vi "Prueba Trip Gap.vi"(11 "Class 2.lvclass":refnum<class "Class 2.lvclass">) -> (3 "Class 2.lvclass 2":refnum<class "Class 2.lvclass">)   [LabVIEW 2019, in "Class 2.lvclass"]
uses:
  Class 2.lvclass
  Class 2.lvclass/Class 2.ctl
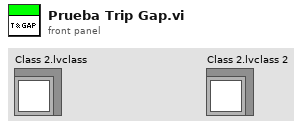
[diagram p1: front panel]
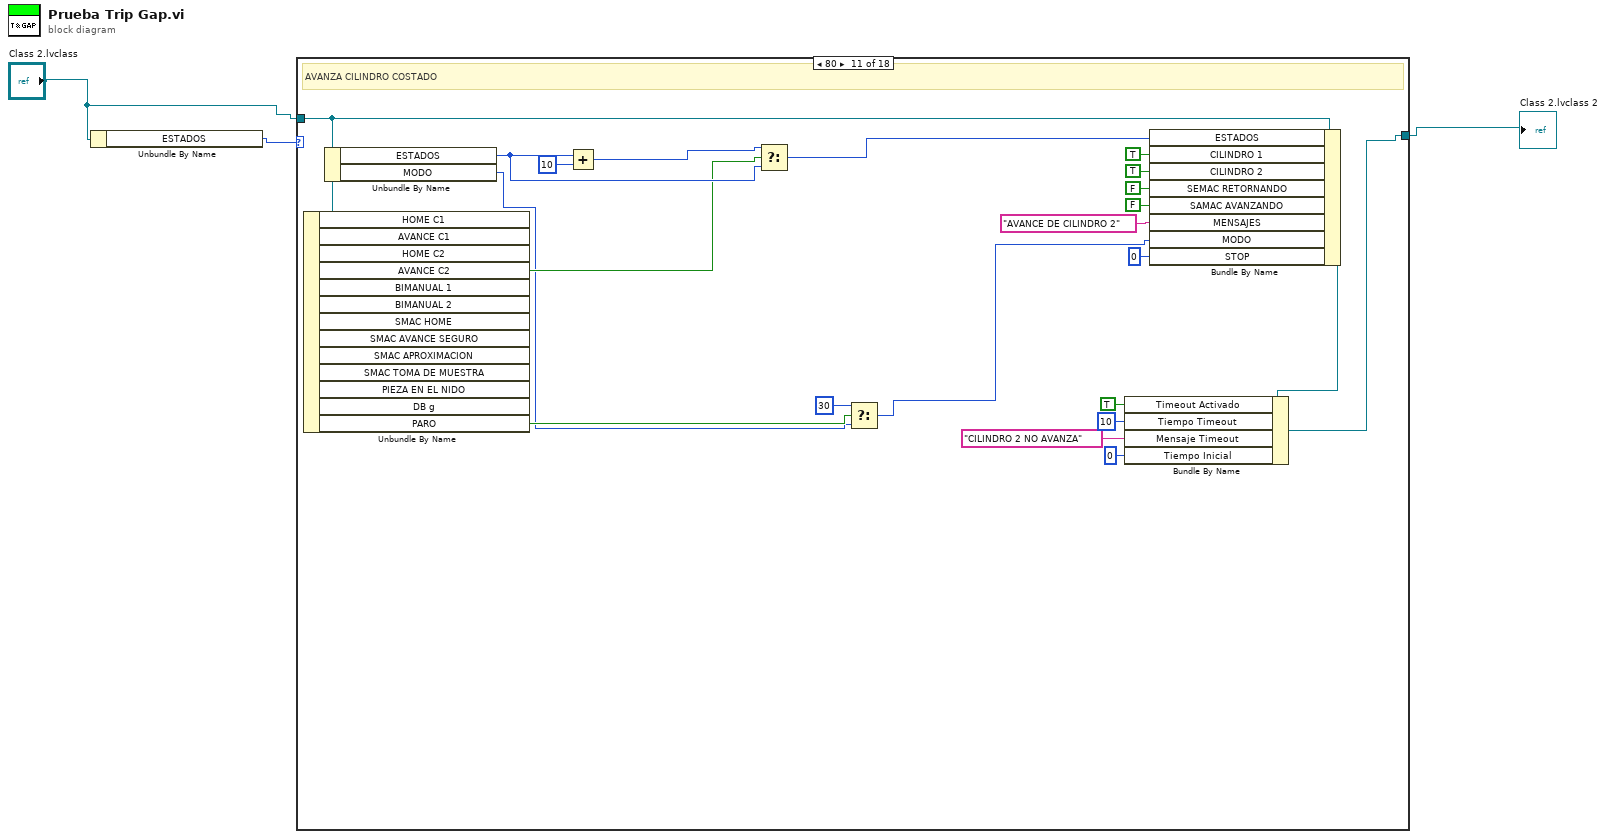
[diagram p0: block diagram]
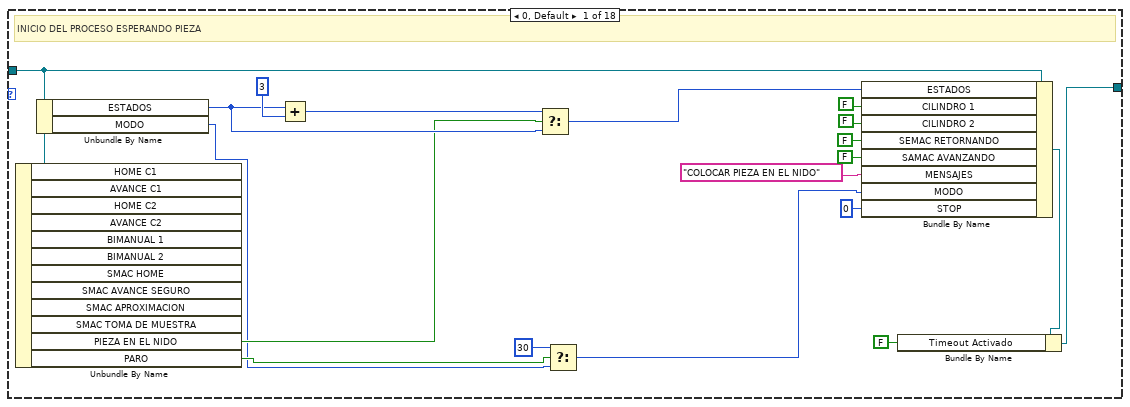
[diagram p2: hidden frame]
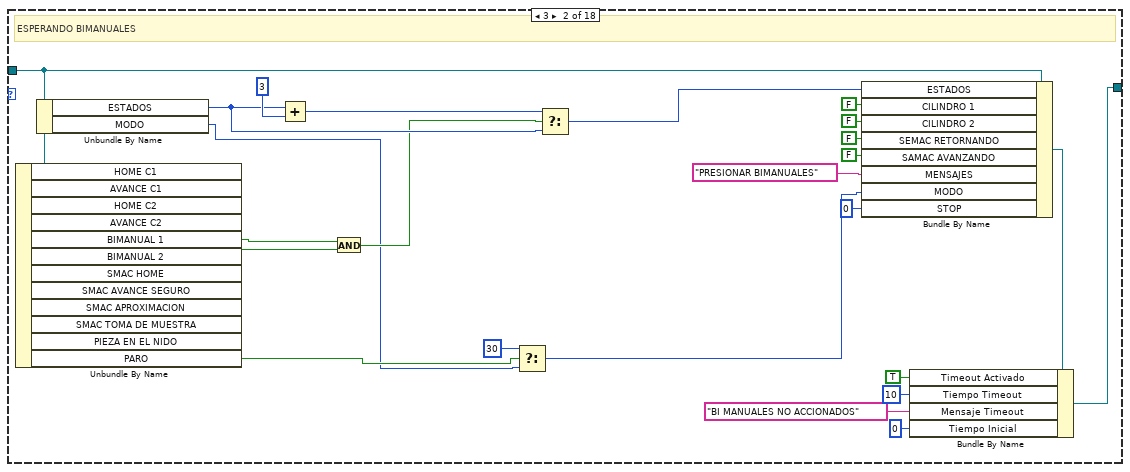
[diagram p3: hidden frame]
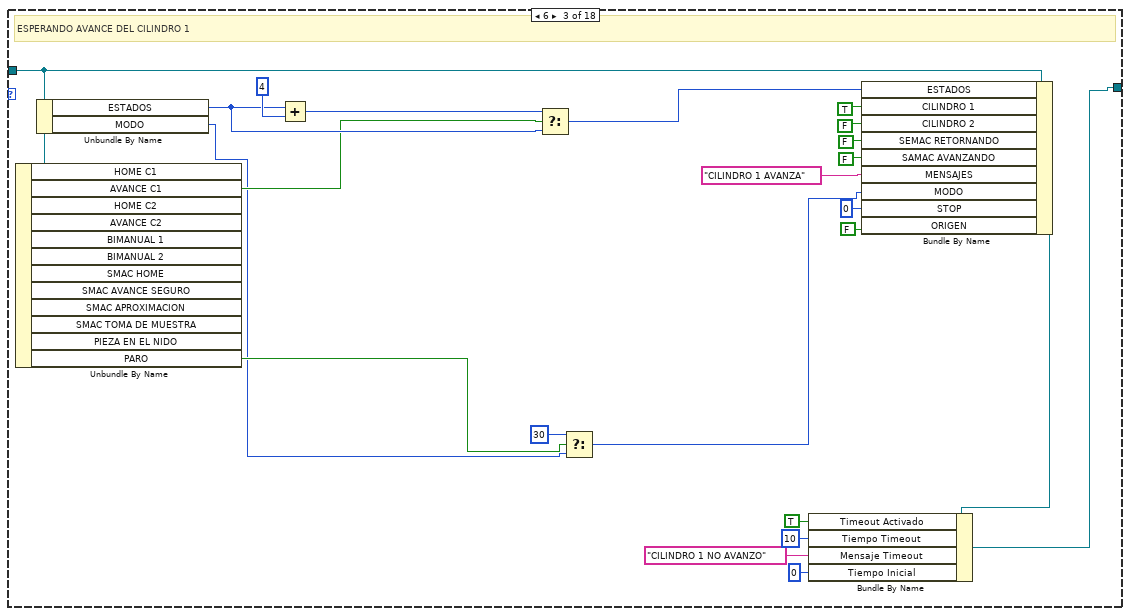
[diagram p4: hidden frame]
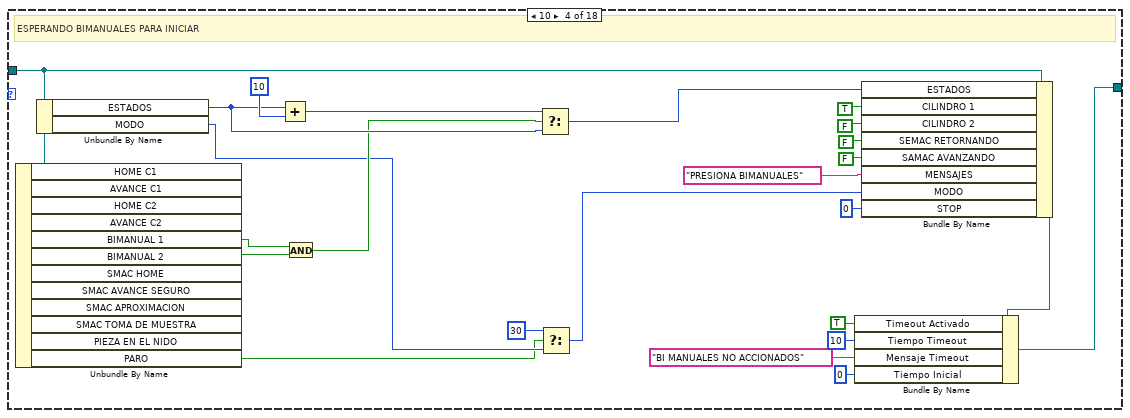
[diagram p5: hidden frame]
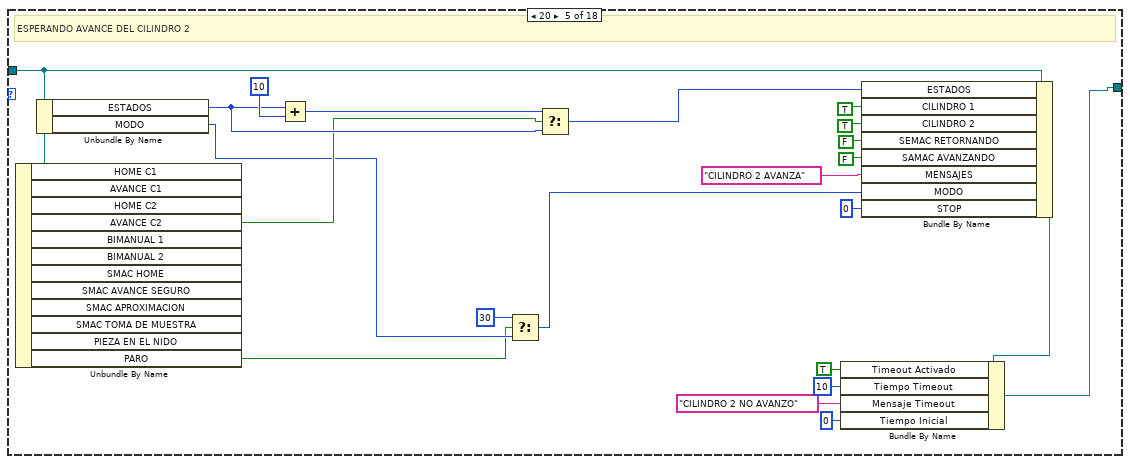
[diagram p6: hidden frame]
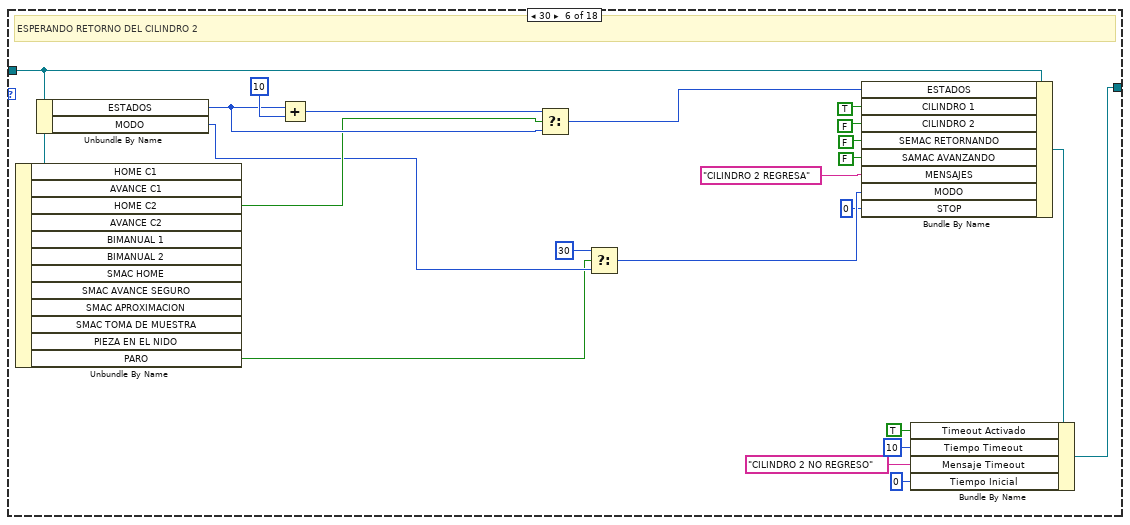
[diagram p7: hidden frame]
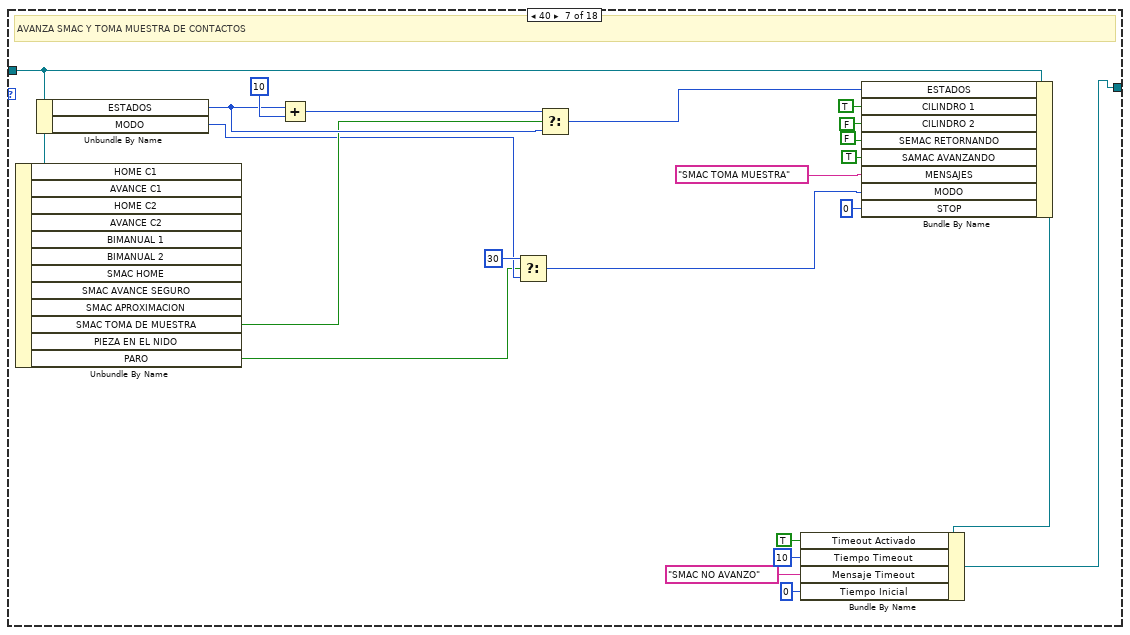
[diagram p8: hidden frame]
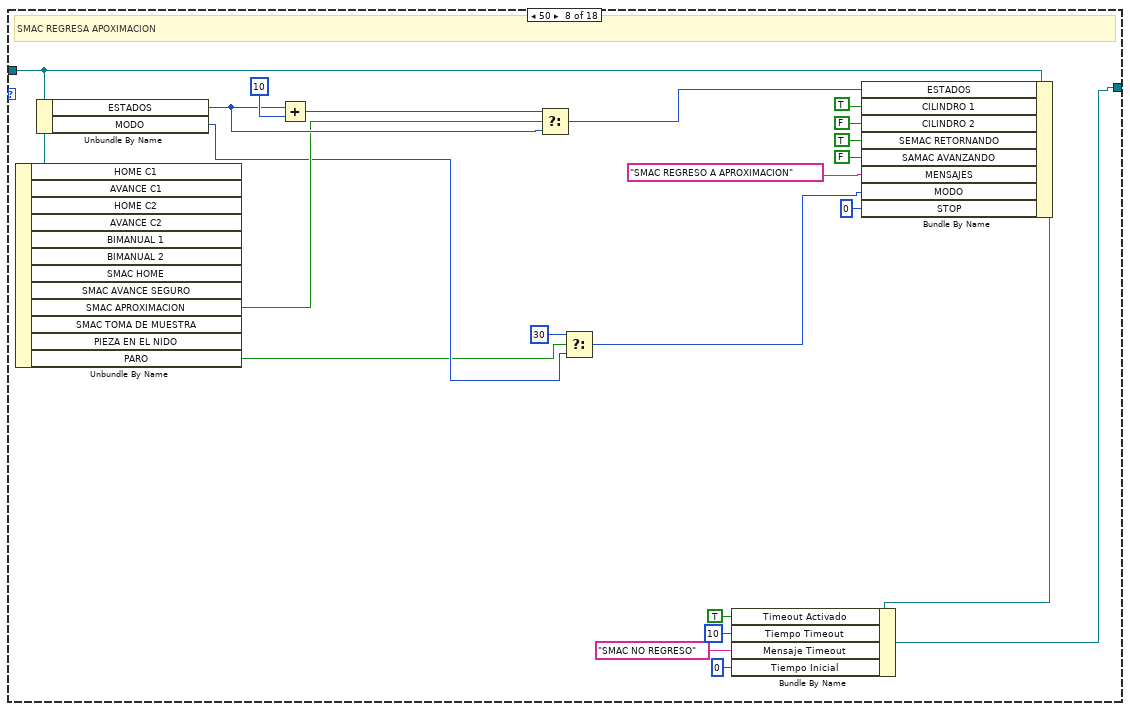
[diagram p9: hidden frame]
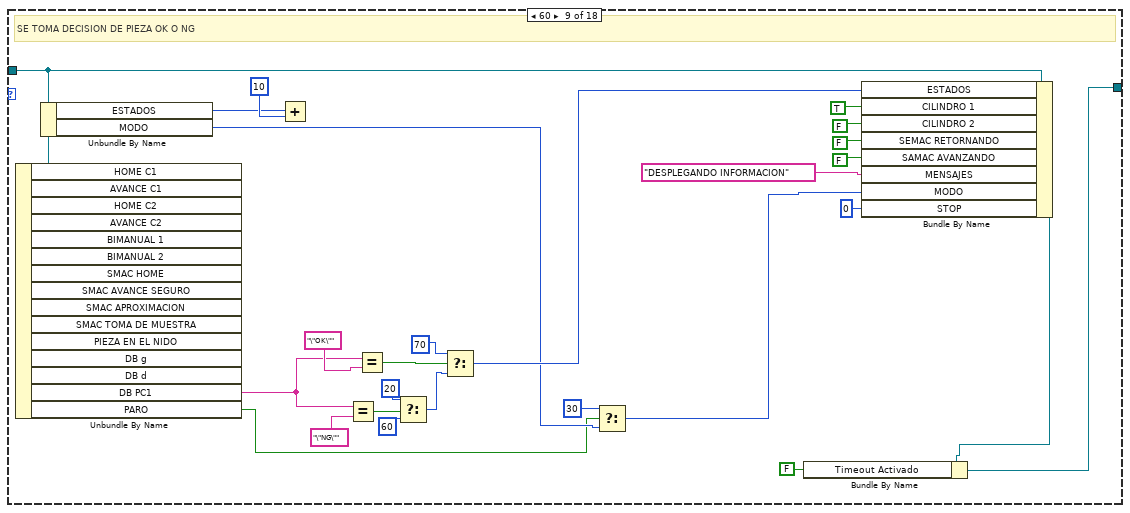
[diagram p10: hidden frame]
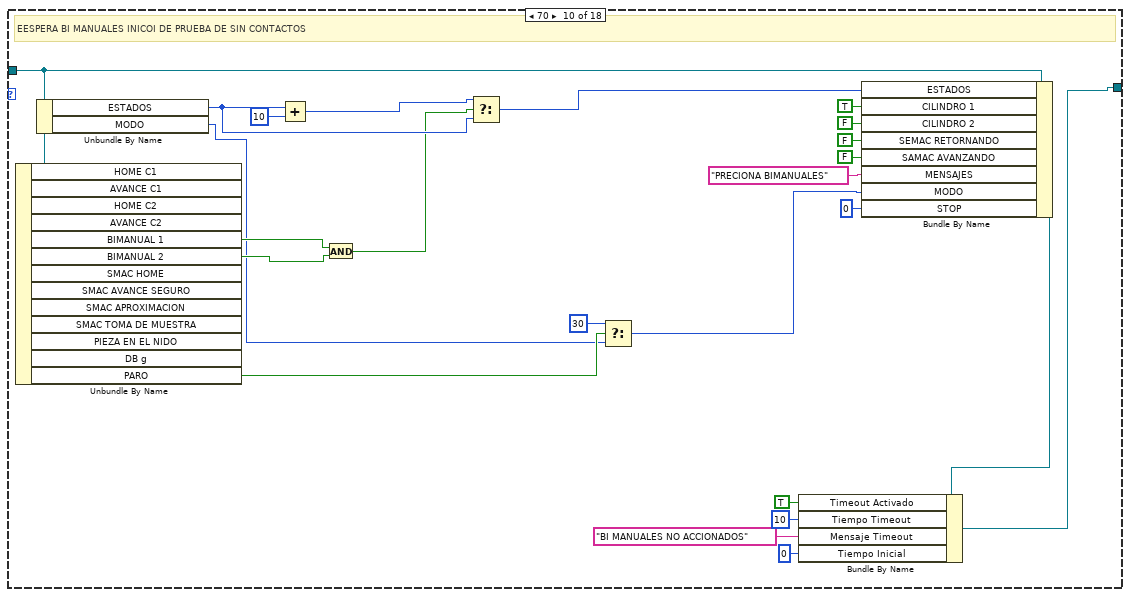
[diagram p11: hidden frame]
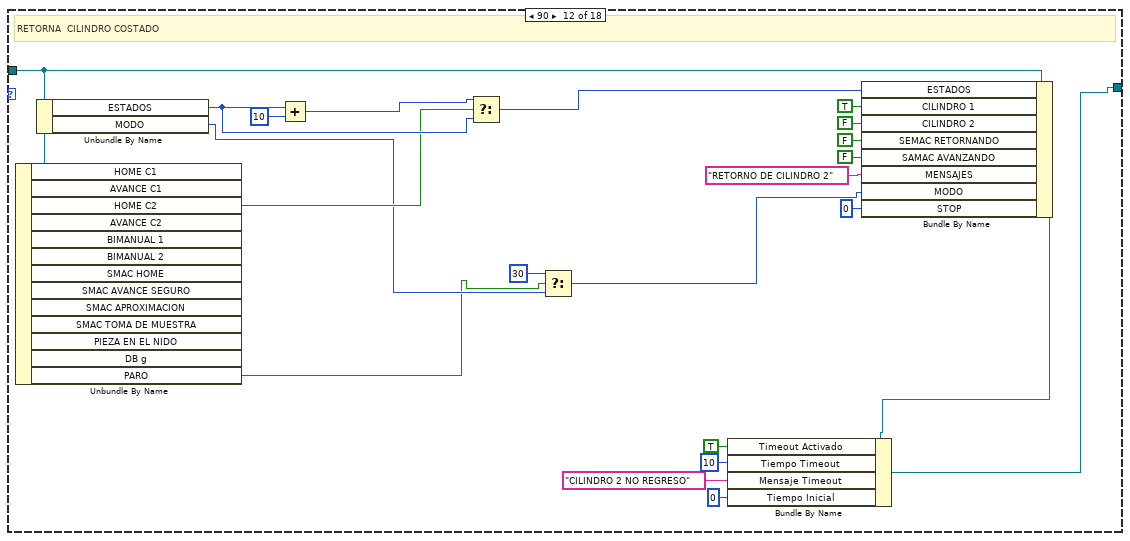
[diagram p12: hidden frame]
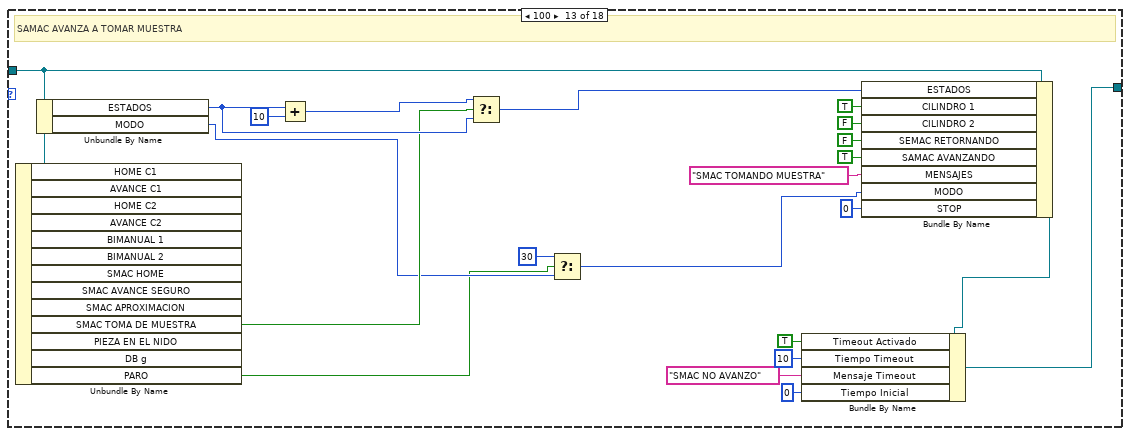
[diagram p13: hidden frame]
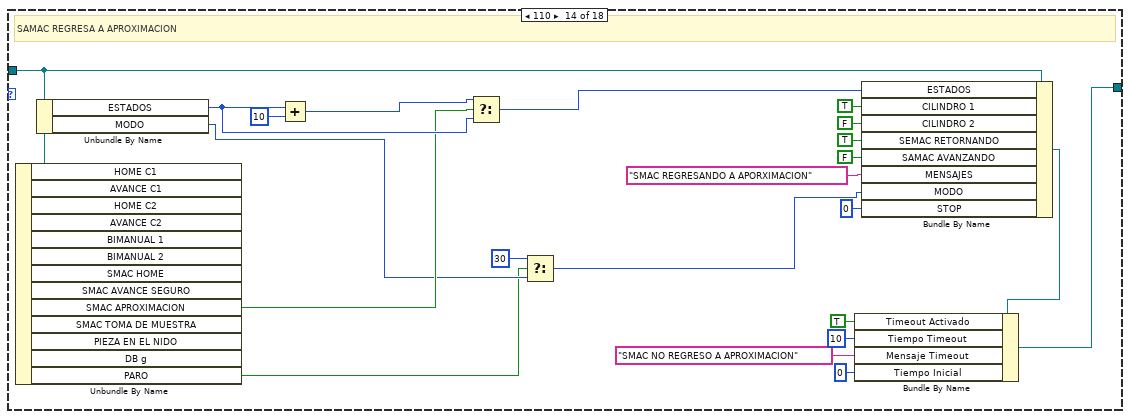
[diagram p14: hidden frame]
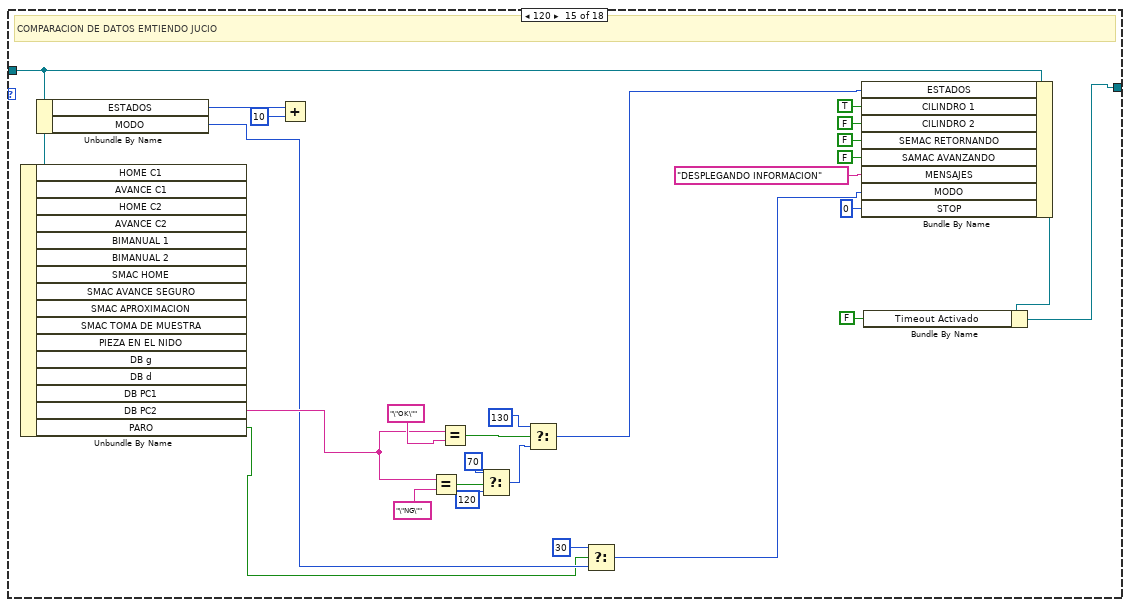
[diagram p15: hidden frame]
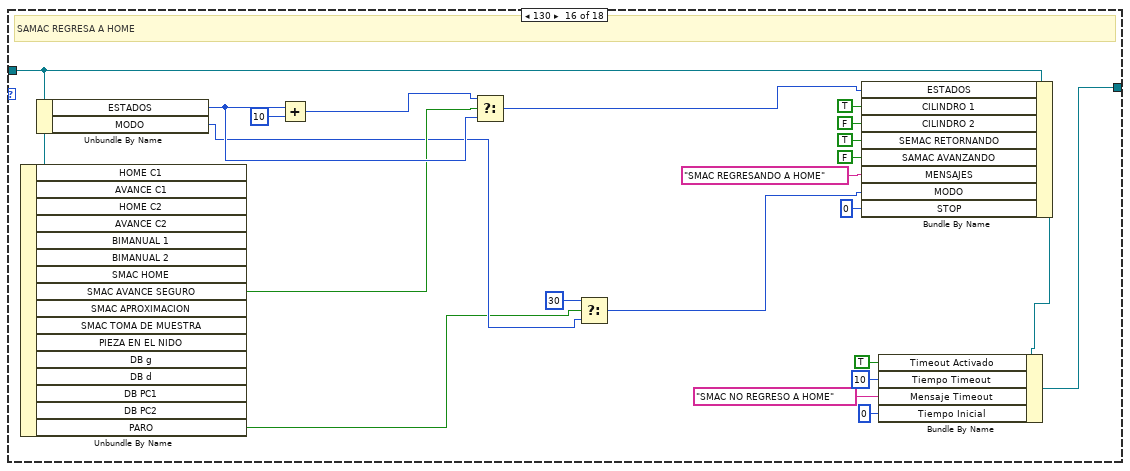
[diagram p16: hidden frame]
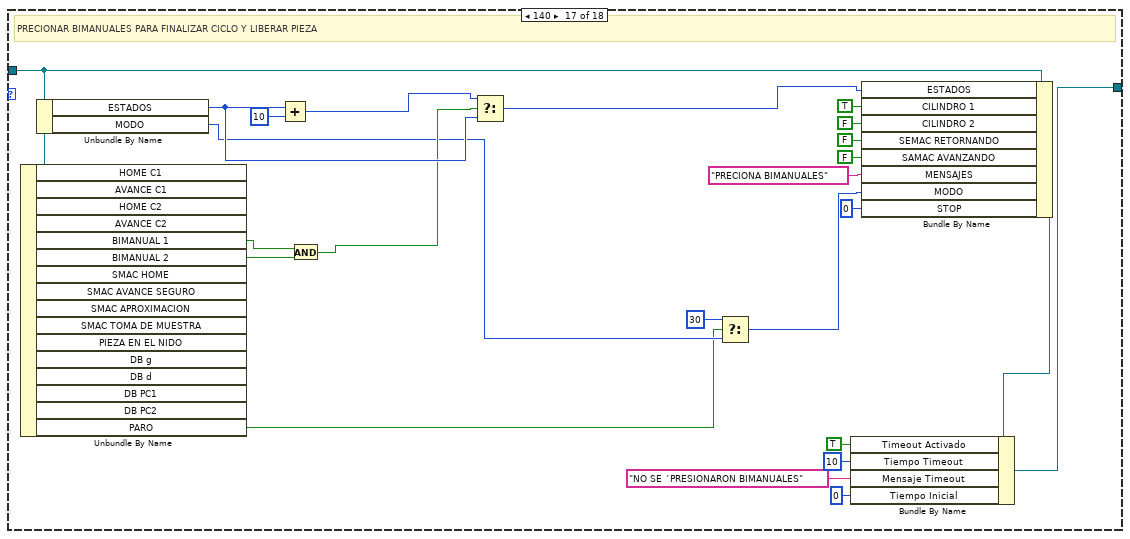
[diagram p17: hidden frame]
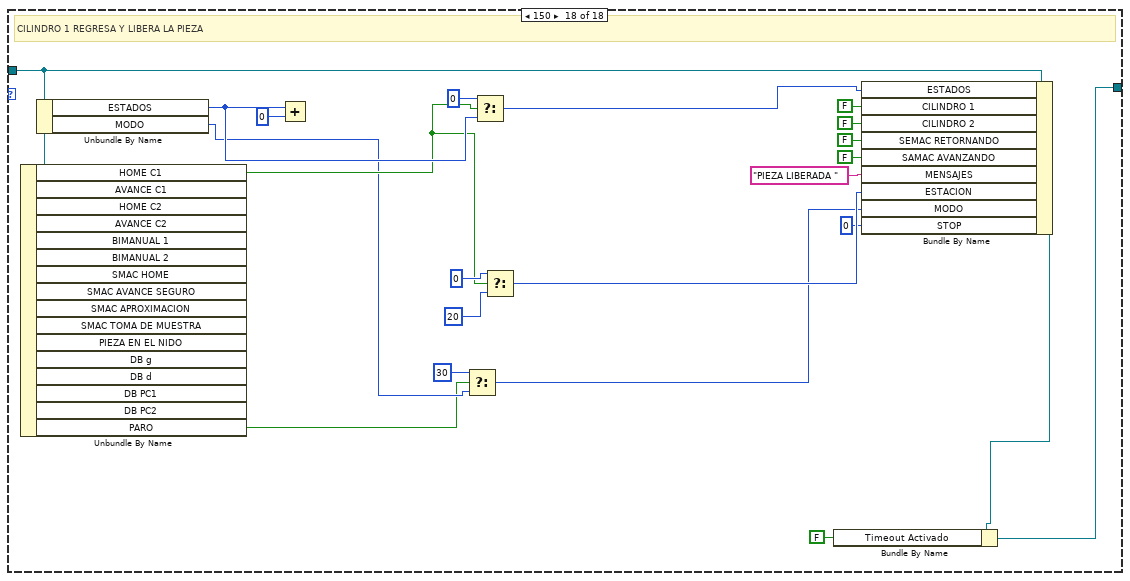
[diagram p18: hidden frame]
diagram:
  n1 = Unbundle By Name("Class 2.lvclass") -> ("ESTADOS"=w3:i16)
  n2 = case shown="80" w3 {
    tunnel: "Class 2.lvclass" -> [w18 w42 w65 w89 w111 w133 w155 w177 w206 w230 w252 w274 w296 w318 w344 w366 w390 w412]
    tunnel: [w4 w23 w47 w70 w94 w116 w138 w160 w182 w208 w232 w254 w276 w298 w320 w346 w368 w392] -> w1
    frame 0, Default {
      # "INICIO DEL PROCESO ESPERANDO PIEZA"
      n3 = Unbundle By Name(w18) -> ("PIEZA EN EL NIDO"=w16:bool, "PARO"=w8:bool)  [unwired: 10 out]
      n4 = Unbundle By Name(w18) -> ("ESTADOS"=w20:i16, "MODO"=w7:i16)
      n5 = Add(x=w20, y=i16 3) -> (x+y=w21:i16)
      n6 = Select(t=w21, s=w16, f=w20) -> (s? t:f=w19:i16)
      n7 = Select(t=i16 30, s=w8, f=w7) -> (s? t:f=w10:i16)
      n8 = Bundle By Name(cluster=w18, "ESTADOS"=w19, "CILINDRO 1"=FALSE ("SALIDAS.CILINDRO 1"), "CILINDRO 2"=FALSE ("SALIDAS.CILINDRO 2"), "SEMAC RETORNANDO"=FALSE ("SALIDAS.SEMAC RETORNANDO"), "SAMAC AVANZANDO"=FALSE ("SALIDAS.SAMAC AVANZANDO"), "MENSAJES"="COLOCAR PIEZA EN EL NIDO" ("SALIDAS.MENSAJES"), "MODO"=w10, "STOP"=i16 0 ("MAQ DE ESTADOS.STOP")) -> (w5:refnum<class "Class 2.lvclass">)
      n9 = Bundle By Name(cluster=w5, "Timeout Activado"=FALSE ("Timeout.Timeout Activado")) -> (w4:refnum<class "Class 2.lvclass">)
    }
    frame 3 {
      # "ESPERANDO BIMANUALES"
      n10 = Unbundle By Name(w42) -> ("BIMANUAL 1"=w36:bool, "BIMANUAL 2"=w35:bool, "PARO"=w30:bool)  [unwired: 9 out]
      n11 = Unbundle By Name(w42) -> ("ESTADOS"=w44:i16, "MODO"=w29:i16)
      n12 = Add(x=w44, y=i16 3) -> (x+y=w45:i16)
      n13 = And(x=w36, y=w35) -> (x .and. y?=w34:bool)
      n14 = Select(t=i16 30, s=w30, f=w29) -> (s? t:f=w32:i16)
      n15 = Select(t=w45, s=w34, f=w44) -> (s? t:f=w43:i16)
      n16 = Bundle By Name(cluster=w42, "ESTADOS"=w43, "CILINDRO 1"=FALSE ("SALIDAS.CILINDRO 1"), "CILINDRO 2"=FALSE ("SALIDAS.CILINDRO 2"), "SEMAC RETORNANDO"=FALSE ("SALIDAS.SEMAC RETORNANDO"), "SAMAC AVANZANDO"=FALSE ("SALIDAS.SAMAC AVANZANDO"), "MENSAJES"="PRESIONAR BIMANUALES" ("SALIDAS.MENSAJES"), "MODO"=w32, "STOP"=i16 0 ("MAQ DE ESTADOS.STOP")) -> (w24:refnum<class "Class 2.lvclass">)
      n17 = Bundle By Name(cluster=w24, "Timeout Activado"=TRUE ("Timeout.Timeout Activado"), "Tiempo Timeout"=u32 10 ("Timeout.Tiempo Timeout"), "Mensaje Timeout"="BI MANUALES NO ACCIONADOS" ("Timeout.Mensaje Timeout"), "Tiempo Inicial"=u32 0 ("Timeout.Tiempo Inicial")) -> (w23:refnum<class "Class 2.lvclass">)
    }
    frame 6 {
      # "ESPERANDO AVANCE DEL CILINDRO 1"
      n18 = Unbundle By Name(w65) -> ("AVANCE C1"=w59:bool, "PARO"=w55:bool)  [unwired: 10 out]
      n19 = Unbundle By Name(w65) -> ("ESTADOS"=w67:i16, "MODO"=w54:i16)
      n20 = Add(x=w67, y=i16 4) -> (x+y=w68:i16)
      n21 = Select(t=w68, s=w59, f=w67) -> (s? t:f=w66:i16)
      n22 = Select(t=i16 30, s=w55, f=w54) -> (s? t:f=w57:i16)
      n23 = Bundle By Name(cluster=w65, "ESTADOS"=w66, "CILINDRO 1"=TRUE ("SALIDAS.CILINDRO 1"), "CILINDRO 2"=FALSE ("SALIDAS.CILINDRO 2"), "SEMAC RETORNANDO"=FALSE ("SALIDAS.SEMAC RETORNANDO"), "SAMAC AVANZANDO"=FALSE ("SALIDAS.SAMAC AVANZANDO"), "MENSAJES"="CILINDRO 1 AVANZA" ("SALIDAS.MENSAJES"), "MODO"=w57, "STOP"=i16 0 ("MAQ DE ESTADOS.STOP"), "ORIGEN"=FALSE ("PROCESO.ORIGEN")) -> (w48:refnum<class "Class 2.lvclass">)
      n24 = Bundle By Name(cluster=w48, "Timeout Activado"=TRUE ("Timeout.Timeout Activado"), "Tiempo Timeout"=u32 10 ("Timeout.Tiempo Timeout"), "Mensaje Timeout"="CILINDRO 1 NO AVANZO" ("Timeout.Mensaje Timeout"), "Tiempo Inicial"=u32 0 ("Timeout.Tiempo Inicial")) -> (w47:refnum<class "Class 2.lvclass">)
    }
    frame 10 {
      # "ESPERANDO BIMANUALES PARA INICIAR"
      n25 = Unbundle By Name(w89) -> ("BIMANUAL 1"=w83:bool, "BIMANUAL 2"=w82:bool, "PARO"=w76:bool)  [unwired: 9 out]
      n26 = Unbundle By Name(w89) -> ("ESTADOS"=w91:i16, "MODO"=w77:i16)
      n27 = Add(x=w91, y=i16 10) -> (x+y=w92:i16)
      n28 = And(x=w83, y=w82) -> (x .and. y?=w81:bool)
      n29 = Select(t=w92, s=w81, f=w91) -> (s? t:f=w90:i16)
      n30 = Select(t=i16 30, s=w76, f=w77) -> (s? t:f=w79:i16)
      n31 = Bundle By Name(cluster=w89, "ESTADOS"=w90, "CILINDRO 1"=TRUE ("SALIDAS.CILINDRO 1"), "CILINDRO 2"=FALSE ("SALIDAS.CILINDRO 2"), "SEMAC RETORNANDO"=FALSE ("SALIDAS.SEMAC RETORNANDO"), "SAMAC AVANZANDO"=FALSE ("SALIDAS.SAMAC AVANZANDO"), "MENSAJES"="PRESIONA BIMANUALES" ("SALIDAS.MENSAJES"), "MODO"=w79, "STOP"=i16 0 ("MAQ DE ESTADOS.STOP")) -> (w71:refnum<class "Class 2.lvclass">)
      n32 = Bundle By Name(cluster=w71, "Timeout Activado"=TRUE ("Timeout.Timeout Activado"), "Tiempo Timeout"=u32 10 ("Timeout.Tiempo Timeout"), "Mensaje Timeout"="BI MANUALES NO ACCIONADOS" ("Timeout.Mensaje Timeout"), "Tiempo Inicial"=u32 0 ("Timeout.Tiempo Inicial")) -> (w70:refnum<class "Class 2.lvclass">)
    }
    frame 20 {
      # "ESPERANDO AVANCE DEL CILINDRO 2"
      n33 = Unbundle By Name(w111) -> ("AVANCE C2"=w105:bool, "PARO"=w100:bool)  [unwired: 10 out]
      n34 = Unbundle By Name(w111) -> ("ESTADOS"=w113:i16, "MODO"=w101:i16)
      n35 = Add(x=w113, y=i16 10) -> (x+y=w114:i16)
      n36 = Select(t=i16 30, s=w100, f=w101) -> (s? t:f=w103:i16)
      n37 = Select(t=w114, s=w105, f=w113) -> (s? t:f=w112:i16)
      n38 = Bundle By Name(cluster=w111, "ESTADOS"=w112, "CILINDRO 1"=TRUE ("SALIDAS.CILINDRO 1"), "CILINDRO 2"=TRUE ("SALIDAS.CILINDRO 2"), "SEMAC RETORNANDO"=FALSE ("SALIDAS.SEMAC RETORNANDO"), "SAMAC AVANZANDO"=FALSE ("SALIDAS.SAMAC AVANZANDO"), "MENSAJES"="CILINDRO 2 AVANZA" ("SALIDAS.MENSAJES"), "MODO"=w103, "STOP"=i16 0 ("MAQ DE ESTADOS.STOP")) -> (w95:refnum<class "Class 2.lvclass">)
      n39 = Bundle By Name(cluster=w95, "Timeout Activado"=TRUE ("Timeout.Timeout Activado"), "Tiempo Timeout"=u32 10 ("Timeout.Tiempo Timeout"), "Mensaje Timeout"="CILINDRO 2 NO AVANZO" ("Timeout.Mensaje Timeout"), "Tiempo Inicial"=u32 0 ("Timeout.Tiempo Inicial")) -> (w94:refnum<class "Class 2.lvclass">)
    }
    frame 30 {
      # "ESPERANDO RETORNO DEL CILINDRO 2"
      n40 = Unbundle By Name(w133) -> ("HOME C2"=w127:bool, "PARO"=w122:bool)  [unwired: 10 out]
      n41 = Unbundle By Name(w133) -> ("ESTADOS"=w135:i16, "MODO"=w123:i16)
      n42 = Add(x=w135, y=i16 10) -> (x+y=w136:i16)
      n43 = Select(t=w136, s=w127, f=w135) -> (s? t:f=w134:i16)
      n44 = Select(t=i16 30, s=w122, f=w123) -> (s? t:f=w125:i16)
      n45 = Bundle By Name(cluster=w133, "ESTADOS"=w134, "CILINDRO 1"=TRUE ("SALIDAS.CILINDRO 1"), "CILINDRO 2"=FALSE ("SALIDAS.CILINDRO 2"), "SEMAC RETORNANDO"=FALSE ("SALIDAS.SEMAC RETORNANDO"), "SAMAC AVANZANDO"=FALSE ("SALIDAS.SAMAC AVANZANDO"), "MENSAJES"="CILINDRO 2 REGRESA" ("SALIDAS.MENSAJES"), "MODO"=w125, "STOP"=i16 0 ("MAQ DE ESTADOS.STOP")) -> (w117:refnum<class "Class 2.lvclass">)
      n46 = Bundle By Name(cluster=w117, "Timeout Activado"=TRUE ("Timeout.Timeout Activado"), "Tiempo Timeout"=u32 10 ("Timeout.Tiempo Timeout"), "Mensaje Timeout"="CILINDRO 2 NO REGRESO" ("Timeout.Mensaje Timeout"), "Tiempo Inicial"=u32 0 ("Timeout.Tiempo Inicial")) -> (w116:refnum<class "Class 2.lvclass">)
    }
    frame 40 {
      # "AVANZA SMAC Y TOMA MUESTRA DE CONTACTOS"
      n47 = Unbundle By Name(w155) -> ("SMAC TOMA DE MUESTRA"=w149:bool, "PARO"=w144:bool)  [unwired: 10 out]
      n48 = Unbundle By Name(w155) -> ("ESTADOS"=w157:i16, "MODO"=w145:i16)
      n49 = Add(x=w157, y=i16 10) -> (x+y=w158:i16)
      n50 = Select(t=i16 30, s=w144, f=w145) -> (s? t:f=w147:i16)
      n51 = Select(t=w158, s=w149, f=w157) -> (s? t:f=w156:i16)
      n52 = Bundle By Name(cluster=w155, "ESTADOS"=w156, "CILINDRO 1"=TRUE ("SALIDAS.CILINDRO 1"), "CILINDRO 2"=FALSE ("SALIDAS.CILINDRO 2"), "SEMAC RETORNANDO"=FALSE ("SALIDAS.SEMAC RETORNANDO"), "SAMAC AVANZANDO"=TRUE ("SALIDAS.SAMAC AVANZANDO"), "MENSAJES"="SMAC TOMA MUESTRA" ("SALIDAS.MENSAJES"), "MODO"=w147, "STOP"=i16 0 ("MAQ DE ESTADOS.STOP")) -> (w139:refnum<class "Class 2.lvclass">)
      n53 = Bundle By Name(cluster=w139, "Timeout Activado"=TRUE ("Timeout.Timeout Activado"), "Tiempo Timeout"=u32 10 ("Timeout.Tiempo Timeout"), "Mensaje Timeout"="SMAC NO AVANZO" ("Timeout.Mensaje Timeout"), "Tiempo Inicial"=u32 0 ("Timeout.Tiempo Inicial")) -> (w138:refnum<class "Class 2.lvclass">)
    }
    frame 50 {
      # "SMAC REGRESA APOXIMACION"
      n54 = Unbundle By Name(w177) -> ("SMAC APROXIMACION"=w171:bool, "PARO"=w166:bool)  [unwired: 10 out]
      n55 = Unbundle By Name(w177) -> ("ESTADOS"=w179:i16, "MODO"=w167:i16)
      n56 = Add(x=w179, y=i16 10) -> (x+y=w180:i16)
      n57 = Select(t=w180, s=w171, f=w179) -> (s? t:f=w178:i16)
      n58 = Select(t=i16 30, s=w166, f=w167) -> (s? t:f=w169:i16)
      n59 = Bundle By Name(cluster=w177, "ESTADOS"=w178, "CILINDRO 1"=TRUE ("SALIDAS.CILINDRO 1"), "CILINDRO 2"=FALSE ("SALIDAS.CILINDRO 2"), "SEMAC RETORNANDO"=TRUE ("SALIDAS.SEMAC RETORNANDO"), "SAMAC AVANZANDO"=FALSE ("SALIDAS.SAMAC AVANZANDO"), "MENSAJES"="SMAC REGRESO A APROXIMACION" ("SALIDAS.MENSAJES"), "MODO"=w169, "STOP"=i16 0 ("MAQ DE ESTADOS.STOP")) -> (w161:refnum<class "Class 2.lvclass">)
      n60 = Bundle By Name(cluster=w161, "Timeout Activado"=TRUE ("Timeout.Timeout Activado"), "Tiempo Timeout"=u32 10 ("Timeout.Tiempo Timeout"), "Mensaje Timeout"="SMAC NO REGRESO" ("Timeout.Mensaje Timeout"), "Tiempo Inicial"=u32 0 ("Timeout.Tiempo Inicial")) -> (w160:refnum<class "Class 2.lvclass">)
    }
    frame 60 {
      # "SE TOMA DECISION DE PIEZA OK O NG"
      n61 = Unbundle By Name(w206) -> ("DB PC1"=w190:string, "PARO"=w185:bool)  [unwired: 13 out]
      n62 = Unbundle By Name(w206) -> ("ESTADOS"=w199:i16, "MODO"=w186:i16)
      n63 = Add(x=w199, y=i16 10) -> ()  [unwired: 1 out]
      n64 = Equal?(x=w190, y="\"NG\"") -> (x = y?=w197:bool)
      n65 = Equal?(x=w190, y="\"OK\"") -> (x = y?=w198:bool)
      n66 = Select(t=i16 20 ("y"), s=w197, f=i16 60) -> (s? t:f=w194:i16)
      n67 = Select(t=i16 70, s=w198, f=w194) -> (s? t:f=w192:i16)
      n68 = Select(t=i16 30, s=w185, f=w186) -> (s? t:f=w188:i16)
      n69 = Bundle By Name(cluster=w206, "ESTADOS"=w192, "CILINDRO 1"=TRUE ("SALIDAS.CILINDRO 1"), "CILINDRO 2"=FALSE ("SALIDAS.CILINDRO 2"), "SEMAC RETORNANDO"=FALSE ("SALIDAS.SEMAC RETORNANDO"), "SAMAC AVANZANDO"=FALSE ("SALIDAS.SAMAC AVANZANDO"), "MENSAJES"="DESPLEGANDO INFORMACION" ("SALIDAS.MENSAJES"), "MODO"=w188, "STOP"=i16 0 ("MAQ DE ESTADOS.MODO")) -> (w183:refnum<class "Class 2.lvclass">)
      n70 = Bundle By Name(cluster=w183, "Timeout Activado"=FALSE ("Timeout.Timeout Activado")) -> (w182:refnum<class "Class 2.lvclass">)
    }
    frame 70 {
      # "EESPERA BI MANUALES INICOI DE PRUEBA DE SIN CONTACTOS"
      n71 = Unbundle By Name(w230) -> ("BIMANUAL 1"=w221:bool, "BIMANUAL 2"=w220:bool, "PARO"=w217:bool)  [unwired: 10 out]
      n72 = Unbundle By Name(w230) -> ("ESTADOS"=w223:i16, "MODO"=w216:i16)
      n73 = Add(x=w223, y=i16 10) -> (x+y=w222:i16)
      n74 = And(x=w221, y=w220) -> (x .and. y?=w219:bool)
      n75 = Select(t=w222, s=w219, f=w223) -> (s? t:f=w224:i16)
      n76 = Select(t=i16 30, s=w217, f=w216) -> (s? t:f=w215:i16)
      n77 = Bundle By Name(cluster=w230, "ESTADOS"=w224, "CILINDRO 1"=TRUE ("SALIDAS.CILINDRO 1"), "CILINDRO 2"=FALSE ("SALIDAS.CILINDRO 2"), "SEMAC RETORNANDO"=FALSE ("SALIDAS.SEMAC RETORNANDO"), "SAMAC AVANZANDO"=FALSE ("SALIDAS.SAMAC AVANZANDO"), "MENSAJES"="PRECIONA BIMANUALES" ("SALIDAS.MENSAJES"), "MODO"=w215, "STOP"=i16 0 ("MAQ DE ESTADOS.STOP")) -> (w209:refnum<class "Class 2.lvclass">)
      n78 = Bundle By Name(cluster=w209, "Timeout Activado"=TRUE ("Timeout.Timeout Activado"), "Tiempo Timeout"=u32 10 ("Timeout.Tiempo Timeout"), "Mensaje Timeout"="BI MANUALES NO ACCIONADOS" ("Timeout.Mensaje Timeout"), "Tiempo Inicial"=u32 0 ("Timeout.Tiempo Inicial")) -> (w208:refnum<class "Class 2.lvclass">)
    }
    frame 80 {
      # "AVANZA CILINDRO COSTADO"
      n79 = Unbundle By Name(w252) -> ("AVANCE C2"=w243:bool, "PARO"=w241:bool)  [unwired: 11 out]
      n80 = Unbundle By Name(w252) -> ("ESTADOS"=w245:i16, "MODO"=w240:i16)
      n81 = Add(x=w245, y=i16 10) -> (x+y=w244:i16)
      n82 = Select(t=w244, s=w243, f=w245) -> (s? t:f=w246:i16)
      n83 = Select(t=i16 30, s=w241, f=w240) -> (s? t:f=w239:i16)
      n84 = Bundle By Name(cluster=w252, "ESTADOS"=w246, "CILINDRO 1"=TRUE ("SALIDAS.CILINDRO 1"), "CILINDRO 2"=TRUE ("SALIDAS.CILINDRO 2"), "SEMAC RETORNANDO"=FALSE ("SALIDAS.SEMAC RETORNANDO"), "SAMAC AVANZANDO"=FALSE ("SALIDAS.SAMAC AVANZANDO"), "MENSAJES"="AVANCE DE CILINDRO 2" ("SALIDAS.MENSAJES"), "MODO"=w239, "STOP"=i16 0 ("MAQ DE ESTADOS.STOP")) -> (w233:refnum<class "Class 2.lvclass">)
      n85 = Bundle By Name(cluster=w233, "Timeout Activado"=TRUE ("Timeout.Timeout Activado"), "Tiempo Timeout"=u32 10 ("Timeout.Tiempo Timeout"), "Mensaje Timeout"="CILINDRO 2 NO AVANZA" ("Timeout.Mensaje Timeout"), "Tiempo Inicial"=u32 0 ("Timeout.Tiempo Inicial")) -> (w232:refnum<class "Class 2.lvclass">)
    }
    frame 90 {
      # "RETORNA  CILINDRO COSTADO"
      n86 = Unbundle By Name(w274) -> ("HOME C2"=w265:bool, "PARO"=w261:bool)  [unwired: 11 out]
      n87 = Unbundle By Name(w274) -> ("ESTADOS"=w267:i16, "MODO"=w262:i16)
      n88 = Add(x=w267, y=i16 10) -> (x+y=w266:i16)
      n89 = Select(t=w266, s=w265, f=w267) -> (s? t:f=w268:i16)
      n90 = Select(t=i16 30, s=w261, f=w262) -> (s? t:f=w263:i16)
      n91 = Bundle By Name(cluster=w274, "ESTADOS"=w268, "CILINDRO 1"=TRUE ("SALIDAS.CILINDRO 1"), "CILINDRO 2"=FALSE ("SALIDAS.CILINDRO 2"), "SEMAC RETORNANDO"=FALSE ("SALIDAS.SEMAC RETORNANDO"), "SAMAC AVANZANDO"=FALSE ("SALIDAS.SAMAC AVANZANDO"), "MENSAJES"="RETORNO DE CILINDRO 2" ("SALIDAS.MENSAJES"), "MODO"=w263, "STOP"=i16 0 ("MAQ DE ESTADOS.STOP")) -> (w255:refnum<class "Class 2.lvclass">)
      n92 = Bundle By Name(cluster=w255, "Timeout Activado"=TRUE ("Timeout.Timeout Activado"), "Tiempo Timeout"=u32 10 ("Timeout.Tiempo Timeout"), "Mensaje Timeout"="CILINDRO 2 NO REGRESO" ("Timeout.Mensaje Timeout"), "Tiempo Inicial"=u32 0 ("Timeout.Tiempo Inicial")) -> (w254:refnum<class "Class 2.lvclass">)
    }
    frame 100 {
      # "SAMAC AVANZA A TOMAR MUESTRA"
      n93 = Unbundle By Name(w296) -> ("SMAC TOMA DE MUESTRA"=w287:bool, "PARO"=w282:bool)  [unwired: 11 out]
      n94 = Unbundle By Name(w296) -> ("ESTADOS"=w289:i16, "MODO"=w283:i16)
      n95 = Add(x=w289, y=i16 10) -> (x+y=w288:i16)
      n96 = Select(t=w288, s=w287, f=w289) -> (s? t:f=w290:i16)
      n97 = Select(t=i16 30, s=w282, f=w283) -> (s? t:f=w285:i16)
      n98 = Bundle By Name(cluster=w296, "ESTADOS"=w290, "CILINDRO 1"=TRUE ("SALIDAS.CILINDRO 1"), "CILINDRO 2"=FALSE ("SALIDAS.CILINDRO 2"), "SEMAC RETORNANDO"=FALSE ("SALIDAS.SEMAC RETORNANDO"), "SAMAC AVANZANDO"=TRUE ("SALIDAS.SAMAC AVANZANDO"), "MENSAJES"="SMAC TOMANDO MUESTRA" ("SALIDAS.MENSAJES"), "MODO"=w285, "STOP"=i16 0 ("MAQ DE ESTADOS.STOP")) -> (w277:refnum<class "Class 2.lvclass">)
      n99 = Bundle By Name(cluster=w277, "Timeout Activado"=TRUE ("Timeout.Timeout Activado"), "Tiempo Timeout"=u32 10 ("Timeout.Tiempo Timeout"), "Mensaje Timeout"="SMAC NO AVANZO" ("Timeout.Mensaje Timeout"), "Tiempo Inicial"=u32 0 ("Timeout.Tiempo Inicial")) -> (w276:refnum<class "Class 2.lvclass">)
    }
    frame 110 {
      # "SAMAC REGRESA A APROXIMACION"
      n100 = Unbundle By Name(w318) -> ("SMAC APROXIMACION"=w309:bool, "PARO"=w304:bool)  [unwired: 11 out]
      n101 = Unbundle By Name(w318) -> ("ESTADOS"=w311:i16, "MODO"=w305:i16)
      n102 = Add(x=w311, y=i16 10) -> (x+y=w310:i16)
      n103 = Select(t=w310, s=w309, f=w311) -> (s? t:f=w312:i16)
      n104 = Select(t=i16 30, s=w304, f=w305) -> (s? t:f=w307:i16)
      n105 = Bundle By Name(cluster=w318, "ESTADOS"=w312, "CILINDRO 1"=TRUE ("SALIDAS.CILINDRO 1"), "CILINDRO 2"=FALSE ("SALIDAS.CILINDRO 2"), "SEMAC RETORNANDO"=TRUE ("SALIDAS.SEMAC RETORNANDO"), "SAMAC AVANZANDO"=FALSE ("SALIDAS.SAMAC AVANZANDO"), "MENSAJES"="SMAC REGRESANDO A APORXIMACION" ("SALIDAS.MENSAJES"), "MODO"=w307, "STOP"=i16 0 ("MAQ DE ESTADOS.STOP")) -> (w299:refnum<class "Class 2.lvclass">)
      n106 = Bundle By Name(cluster=w299, "Timeout Activado"=TRUE ("Timeout.Timeout Activado"), "Tiempo Timeout"=u32 10 ("Timeout.Tiempo Timeout"), "Mensaje Timeout"="SMAC NO REGRESO A APROXIMACION" ("Timeout.Mensaje Timeout"), "Tiempo Inicial"=u32 0 ("Timeout.Tiempo Inicial")) -> (w298:refnum<class "Class 2.lvclass">)
    }
    frame 120 {
      # "COMPARACION DE DATOS EMTIENDO JUCIO"
      n107 = Unbundle By Name(w344) -> ("DB PC2"=w329:string, "PARO"=w323:bool)  [unwired: 14 out]
      n108 = Unbundle By Name(w344) -> ("ESTADOS"=w338:i16, "MODO"=w324:i16)
      n109 = Add(x=w338, y=i16 10) -> ()  [unwired: 1 out]
      n110 = Equal?(x=w329, y="\"NG\"") -> (x = y?=w335:bool)
      n111 = Equal?(x=w329, y="\"OK\"") -> (x = y?=w336:bool)
      n112 = Select(t=i16 70 ("y"), s=w335, f=i16 120) -> (s? t:f=w332:i16)
      n113 = Select(t=i16 130, s=w336, f=w332) -> (s? t:f=w328:i16)
      n114 = Select(t=i16 30, s=w323, f=w324) -> (s? t:f=w326:i16)
      n115 = Bundle By Name(cluster=w344, "ESTADOS"=w328, "CILINDRO 1"=TRUE ("SALIDAS.CILINDRO 1"), "CILINDRO 2"=FALSE ("SALIDAS.CILINDRO 2"), "SEMAC RETORNANDO"=FALSE ("SALIDAS.SEMAC RETORNANDO"), "SAMAC AVANZANDO"=FALSE ("SALIDAS.SAMAC AVANZANDO"), "MENSAJES"="DESPLEGANDO INFORMACION" ("SALIDAS.MENSAJES"), "MODO"=w326, "STOP"=i16 0 ("MAQ DE ESTADOS.STOP")) -> (w321:refnum<class "Class 2.lvclass">)
      n116 = Bundle By Name(cluster=w321, "Timeout Activado"=FALSE ("Timeout.Timeout Activado")) -> (w320:refnum<class "Class 2.lvclass">)
    }
    frame 130 {
      # "SAMAC REGRESA A HOME"
      n117 = Unbundle By Name(w366) -> ("SMAC AVANCE SEGURO"=w357:bool, "PARO"=w352:bool)  [unwired: 14 out]
      n118 = Unbundle By Name(w366) -> ("ESTADOS"=w358:i16, "MODO"=w353:i16)
      n119 = Add(x=w358, y=i16 10) -> (x+y=w359:i16)
      n120 = Select(t=w359, s=w357, f=w358) -> (s? t:f=w360:i16)
      n121 = Select(t=i16 30, s=w352, f=w353) -> (s? t:f=w355:i16)
      n122 = Bundle By Name(cluster=w366, "ESTADOS"=w360, "CILINDRO 1"=TRUE ("SALIDAS.CILINDRO 1"), "CILINDRO 2"=FALSE ("SALIDAS.CILINDRO 2"), "SEMAC RETORNANDO"=TRUE ("SALIDAS.SEMAC RETORNANDO"), "SAMAC AVANZANDO"=FALSE ("SALIDAS.SAMAC AVANZANDO"), "MENSAJES"="SMAC REGRESANDO A HOME" ("SALIDAS.MENSAJES"), "MODO"=w355, "STOP"=i16 0 ("MAQ DE ESTADOS.STOP")) -> (w347:refnum<class "Class 2.lvclass">)
      n123 = Bundle By Name(cluster=w347, "Timeout Activado"=TRUE ("Timeout.Timeout Activado"), "Tiempo Timeout"=u32 10 ("Timeout.Tiempo Timeout"), "Mensaje Timeout"="SMAC NO REGRESO A HOME" ("Timeout.Mensaje Timeout"), "Tiempo Inicial"=u32 0 ("Timeout.Tiempo Inicial")) -> (w346:refnum<class "Class 2.lvclass">)
    }
    frame 140 {
      # "PRECIONAR BIMANUALES PARA FINALIZAR CICLO Y LIBERAR PIEZA"
      n124 = Unbundle By Name(w390) -> ("BIMANUAL 1"=w381:bool, "BIMANUAL 2"=w380:bool, "PARO"=w374:bool)  [unwired: 13 out]
      n125 = Unbundle By Name(w390) -> ("ESTADOS"=w382:i16, "MODO"=w375:i16)
      n126 = Add(x=w382, y=i16 10) -> (x+y=w383:i16)
      n127 = And(x=w381, y=w380) -> (x .and. y?=w379:bool)
      n128 = Select(t=w383, s=w379, f=w382) -> (s? t:f=w384:i16)
      n129 = Select(t=i16 30, s=w374, f=w375) -> (s? t:f=w377:i16)
      n130 = Bundle By Name(cluster=w390, "ESTADOS"=w384, "CILINDRO 1"=TRUE ("SALIDAS.CILINDRO 1"), "CILINDRO 2"=FALSE ("SALIDAS.CILINDRO 2"), "SEMAC RETORNANDO"=FALSE ("SALIDAS.SEMAC RETORNANDO"), "SAMAC AVANZANDO"=FALSE ("SALIDAS.SAMAC AVANZANDO"), "MENSAJES"="PRECIONA BIMANUALES" ("SALIDAS.MENSAJES"), "MODO"=w377, "STOP"=i16 0 ("MAQ DE ESTADOS.STOP")) -> (w369:refnum<class "Class 2.lvclass">)
      n131 = Bundle By Name(cluster=w369, "Timeout Activado"=TRUE ("Timeout.Timeout Activado"), "Tiempo Timeout"=u32 10 ("Timeout.Tiempo Timeout"), "Mensaje Timeout"="NO SE ´PRESIONARON BIMANUALES" ("Timeout.Mensaje Timeout"), "Tiempo Inicial"=u32 0 ("Timeout.Tiempo Inicial")) -> (w368:refnum<class "Class 2.lvclass">)
    }
    frame 150 {
      # "CILINDRO 1 REGRESA Y LIBERA LA PIEZA"
      n132 = Unbundle By Name(w412) -> ("HOME C1"=w400:bool, "PARO"=w395:bool)  [unwired: 14 out]
      n133 = Unbundle By Name(w412) -> ("ESTADOS"=w405:i16, "MODO"=w396:i16)
      n134 = Add(x=w405, y=i16 0) -> ()  [unwired: 1 out]
      n135 = Select(t=i16 30, s=w395, f=w396) -> (s? t:f=w398:i16)
      n136 = Select(t=i16 0, s=w400, f=w405) -> (s? t:f=w406:i16)
      n137 = Select(t=i16 0, s=w400, f=i16 20 ("t")) -> (s? t:f=w401:i16)
      n138 = Bundle By Name(cluster=w412, "ESTADOS"=w406, "CILINDRO 1"=FALSE ("SALIDAS.CILINDRO 1"), "CILINDRO 2"=FALSE ("SALIDAS.CILINDRO 2"), "SEMAC RETORNANDO"=FALSE ("SALIDAS.SEMAC RETORNANDO"), "SAMAC AVANZANDO"=FALSE ("SALIDAS.SAMAC AVANZANDO"), "MENSAJES"="PIEZA LIBERADA " ("SALIDAS.MENSAJES"), "ESTACION"=w401, "MODO"=w398, "STOP"=i16 0 ("MAQ DE ESTADOS.STOP")) -> (w393:refnum<class "Class 2.lvclass">)
      n139 = Bundle By Name(cluster=w393, "Timeout Activado"=FALSE ("Timeout.Timeout Activado")) -> (w392:refnum<class "Class 2.lvclass">)
    }
  }
  "Class 2.lvclass 2" <- w1
